vi "sine^2 ramp.vi"(4 "End Amp.":dbl=1.0 format="%.2f", 5 "samples":i32=8) -> (0 "error":i32, 1 "sine^2 Ramp":dbl[](array[numeric])=[0.0, 0.002451791281132127, 0.035439982326093925, 0.15111842453404034, 0.3736393584903548, 0.6589297841848273, 0.9034206591835512, 1.0] format="%.4f", 2 "sine Ramp":dbl[](array[numeric])=[0.0, 0.04951556604879043, 0.1882550990706332, 0.3887395330218427, 0.6112604669781572, 0.8117449009293667, 0.9504844339512095, 1.0] format="%.4f")   [LabVIEW 2015]
doc: "Generates an array containing a ramp pattern."
uses:
  <vilib>/Analysis/NI_AALBase.lvlib
panel:
  # "sine squared Ramp"
  # "`"
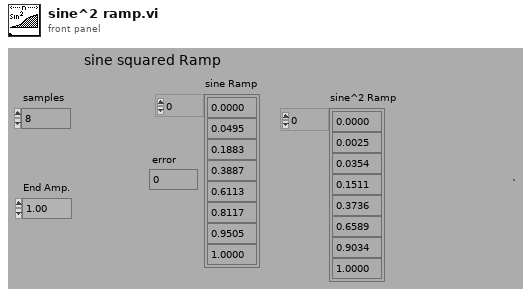
[diagram p1: front panel]
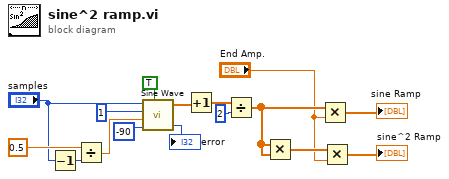
[diagram p0: block diagram]
diagram:
  n1 = Decrement(x="samples") -> (x-1=w11:i32)
  n2 = Divide(x=0.5, y=w11) -> (x/y=w15:dbl)
  n3 = call <vilib>:"Sine Wave.vi"("samples"="samples", "amplitude"=1, "frequency"=w15, "phase in"=-90, "reset phase"=TRUE) -> ("sine wave"=w8:dbl[], "error"=→"error":i32)  [unwired: 1 out]
  n4 = Increment(x=w8) -> (x+1=w7:dbl[])
  n5 = Divide(x=w7, y=2) -> (x/y=w5:dbl[])
  n6 = Multiply(x=w5, y=w5) -> (x*y=w4:dbl[])
  n7 = Multiply(x=w5, y="End Amp.") -> (x*y=→"sine Ramp":dbl[])
  n8 = Multiply(x=w4, y="End Amp.") -> (x*y=→"sine^2 Ramp":dbl[])
